vi "GetLastSelfCalInfo.vi"(8 "error in (no error)":errorcluster, 10 "gRPCid":T4, 11 "ctet_dmm":T1) -> (0 "error out":errorcluster, 3 "ctet_dmm out":T1)   [LabVIEW 2019, in "ctet_dmm User Library.lvlib"]
uses:
  ctet_dmm User Library.lvlib
  Servers/ctet_dmm/gRPC lvSupport/Server API/typeDefs/grpcId.ctl
  Types/ctet_dmm.ctl
  Servers/ctet_dmm/ctet_dmm Class/RPC Messages/measurementservice_DMMConfigResponse/measurementservice_DMMConfigResponse_Data.ctl
  Servers/ctet_dmm/ctet_dmm Class/RPC Messages/measurementservice_ErrorOut/measurementservice_ErrorOut_Data.ctl
  <instrlib>/niDMM/nidmm.llb/niDMM Cal Type.ctl
  Servers/ctet_dmm/ctet_dmm Class/RPC Messages/measurementservice_DMMLastSelfCalInfoResponse/measurementservice_DMMLastSelfCalInfoResponse_Data.ctl
  Servers/ctet_dmm/ctet_dmm Class/ctet_dmm.lvclass
  Servers/ctet_dmm/gRPC lvSupport/gprc-lvsupport.lvlib
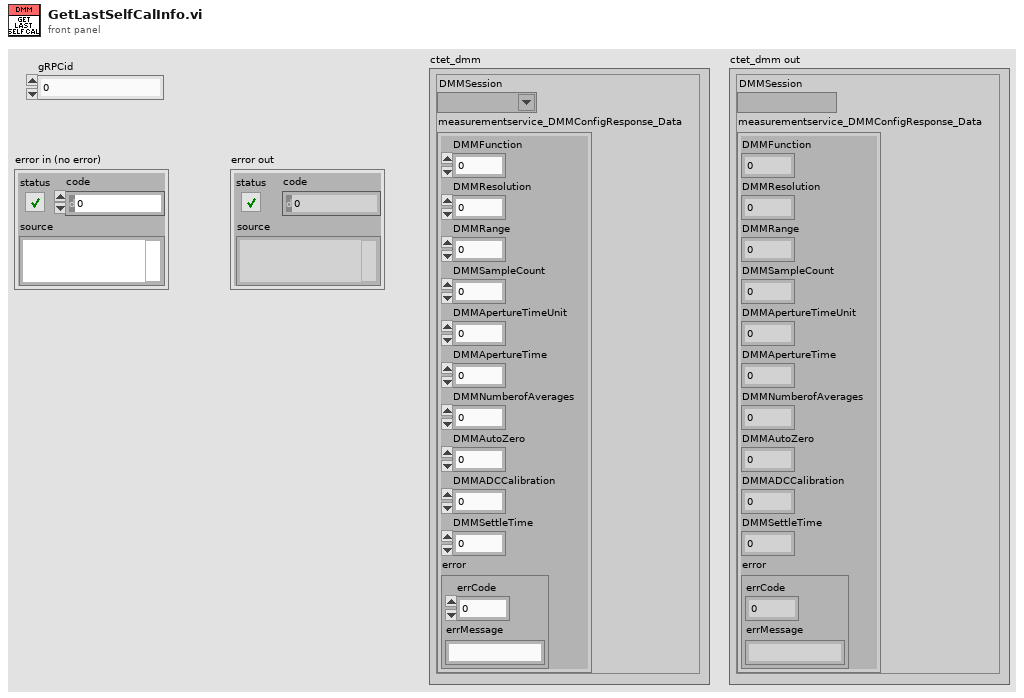
[diagram p1: front panel]
types:
  T1 = typedef "ctet_dmm User Library.lvlib/ctet_dmm.ctl" = cluster{"DMMSession":refnum<k15>, "measurementservice_DMMConfigResponse_Data":T2}
  T2 = typedef "ctet_dmm.lvlib/ctet_dmm.lvclass/measurementservice_DMMConfigResponse_Data.ctl" = cluster{"DMMFunction":i64, "DMMResolution":dbl, "DMMRange":dbl, "DMMSampleCount":i64, "DMMApertureTimeUnit":i64, "DMMApertureTime":dbl, "DMMNumberofAverages":i64, "DMMAutoZero":i64, "DMMADCCalibration":i64, "DMMSettleTime":dbl, "error":T3}
  T3 = typedef "ctet_dmm.lvlib/ctet_dmm.lvclass/measurementservice_ErrorOut_Data.ctl" = cluster{"errCode":i64, "errMessage":string}
  T4 = typedef "ctet_dmm.lvlib/gprc-lvsupport.lvlib/grpcId.ctl" = u64
  T5 = typedef "ctet_dmm.lvlib/ctet_dmm.lvclass/measurementservice_DMMLastSelfCalInfoResponse_Data.ctl" = cluster{"month":i64, "day":i64, "year":i64, "hour":i64, "minute":i64, "error":T3}
  T6 = typedef "niDMM Cal Type.ctl" = enum16{"Internal", "External"}
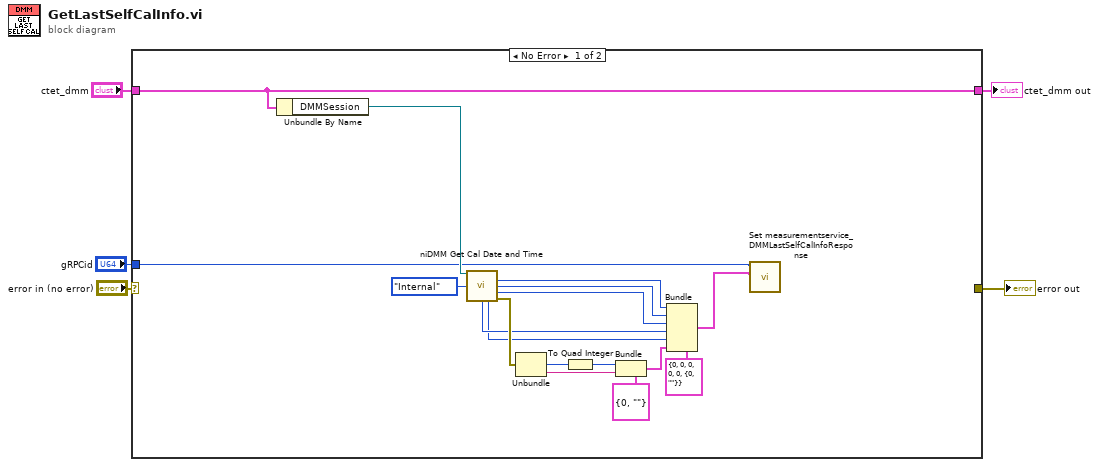
[diagram p0: block diagram]
diagram:
  n1 = case shown="No Error" "error in (no error)" {
    selector: "error in (no error)" -> [_ w24]
    tunnel: [_ w24] -> w5
    tunnel: "gRPCid" -> [w10 _]
    tunnel: "ctet_dmm" -> [w17 w23]
    tunnel: [w17 w23] -> w1
    frame No Error {
      n2 = Unbundle By Name(w17) -> ("DMMSession"=w18:refnum<k15>)
      n3 = call <instrlib>:"niDMM Get Cal Date and Time.vi"("instrument handle"=w18, "Cal Type"=niDMM_Cal_Type."Internal") -> ("Month"=w15:i32, "Day"=w14:i32, "Year"=w13:i32, "Hour"=w12:i32, "Minute"=w11:i32, "error out"=w22:errorcluster)  [unwired: 7 in, 1 out]
      n4 = Unbundle(w22) -> ("code"=w20:i32, "source"=w21:string)  [unwired: 1 out]
      n5 = To Quad Integer(1:w20) -> (0:w19:i64)
      n6 = Bundle(cluster=T3 {"errCode"=0, "errMessage"=""} ("error"), "errCode"=w19, "errMessage"=w21) -> (w6:T3)
      n7 = Bundle(cluster=T5 {"month"=0, "day"=0, "year"=0, "hour"=0, "minute"=0, "error"={"errCode"=0, "errMessage"=""}} ("measurementservice_DMMLastSelfCalInfoResponse_Data"), "month"=w15, "day"=w14, "year"=w13, "hour"=w12, "minute"=w11, "error"=w6) -> (w9:T5)
      n8 = call "Set measurementservice_DMMLastSelfCalInfoResponse.vi"("Message Data"=w9, "gRPCid"=w10) -> ()  [unwired: 9 in, 1 out]
    }
    frame Error {
    }
  }
  "error out" <- w5
  "ctet_dmm out" <- w1
